vi "SystemActive.vi"(0 "DataCluster":T1) -> (1 "Active":bool, 2 "!Active/Exit":bool, 3 "Exit":bool)   [LabVIEW 2020]
uses:
  DataCluster.ctl
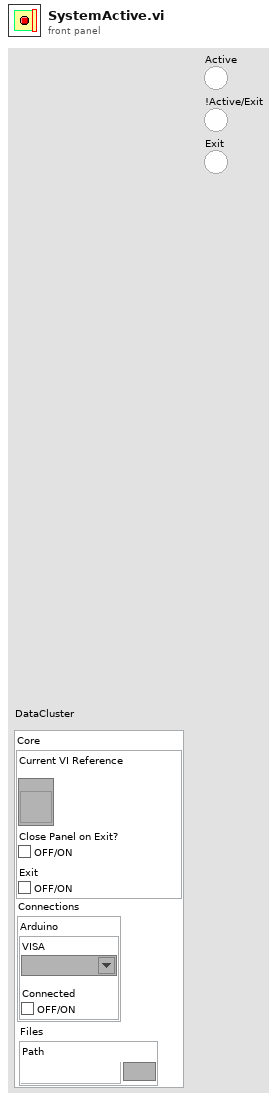
[diagram p1: front panel]
types:
  T1 = typedef "DataCluster.ctl" = cluster{"Core":cluster{"Current VI Reference":refnum<vi>, "Close Panel on Exit?":bool, "Exit":bool}, "Connections":cluster{"Arduino":cluster{"VISA":refnum<visa-resource-name>, "Connected":bool}}, "Files":cluster{"Path":path}}
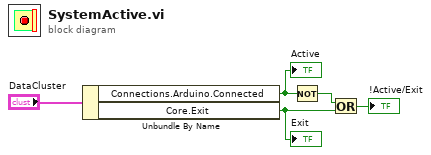
[diagram p0: block diagram]
diagram:
  n1 = Unbundle By Name("DataCluster") -> ("Connections.Arduino.Connected"=w1:bool, "Core.Exit"=w5:bool)
  "Exit" <- w5
  "Active" <- w1
  n2 = Not(x=w1) -> (.not. x?=w4:bool)
  n3 = Or(x=w4, y=w5) -> (x .or. y?=→"!Active/Exit":bool)
